vi "ClientUtilities.vi"(1 "Timout":u8=1, 2 "ServerPort":u16=2402, 3 "ServerName":string="tester") -> (0 "Error":bool)   [LabVIEW 2014]
uses:
  globals/AzCamGlobals.vi
panel:
  out "Count":i32
  # "Trying to connect to AzCamServer, please wait..."
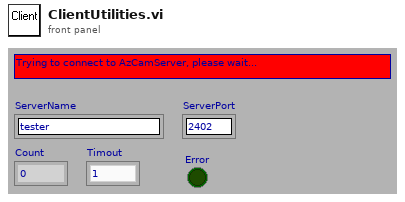
[diagram p1: front panel]
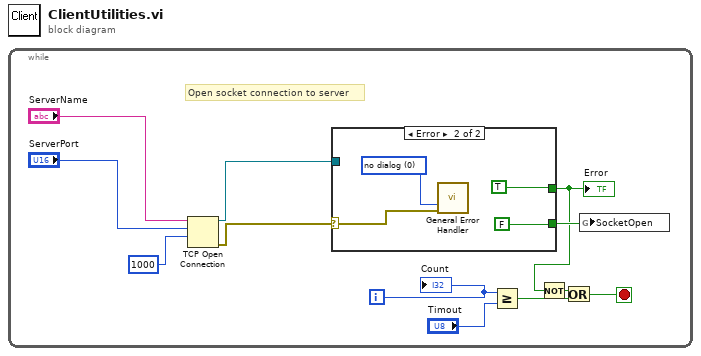
[diagram p0: block diagram]
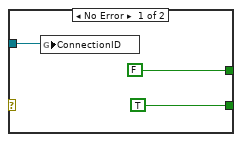
[diagram p2: hidden frame]
diagram:
  n1 = while {
    i -> [w6]
    stop <- w3 stop-if-true
    # "Open socket connection to server"
    n2 = TCP Open Connection(address="ServerName", remote port or service name="ServerPort", timeout ms (60000)=1000) -> (connection ID=w7:refnum<k5>, error out=w9:errorcluster)  [unwired: 2 in]
    n3 = case shown="Error" w9 {
      selector: w9 -> [_ w16]
      tunnel: [FALSE ("Error") TRUE ("Error")] -> w2
      tunnel: [TRUE ("Error") FALSE ("Error")] -> w8
      tunnel: w7 -> [w13 _]
      frame No Error {
        n4 = global write "AzCamGlobals.vi" "ConnectionID"(w13) -> ()
      }
      frame Error {
        w17 = u16 0 items=["no dialog", "OK message", "continue or stop message"] ("type of dialog (OK msg:1)")
        n5 = call <vilib>:"General Error Handler.vi"("type of dialog (OK msg:1)"=w17, "error in (no error)"=w16) -> ()  [unwired: 9 in, 5 out]
      }
    }
    "Error" <- w2
    n6 = Greater Or Equal?(x=w6, y="Timout") -> (x >= y?=w4:bool)
    n7 = Not(x=w2) -> (.not. x?=w1:bool)
    n8 = Or(x=w1, y=w4) -> (x .or. y?=w3:bool)
    n9 = global write "AzCamGlobals.vi" "SocketOpen"(w8) -> ()
    "Count" <- w6
  }
